vi "Ascii to string.vi"(11 "ASCII Code":u8) -> (3 "String":string)   [LabVIEW 2023]
doc: "Converts ascii code to equivalent string"
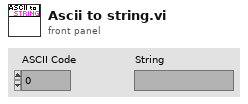
[diagram p1: front panel]
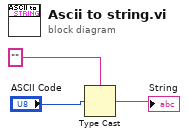
[diagram p0: block diagram]
diagram:
  n1 = Type Cast(type="", x="ASCII Code") -> (*(type *) &x=→"String":string)
